vi "Test App Error Handler is Configured Process Added before Start.vi"(8 "error in (no error)":errorcluster, 11 "Rig Test In":refnum<class "Application Dev Test.lvclass">) -> (0 "error out":errorcluster, 3 "Rig Test Out":refnum<class "Application Dev Test.lvclass">)   [LabVIEW 2020, in "Application Dev Test.lvclass"]
uses:
  Application Dev Test.lvclass
  C:/Program Files (x86)/National Instruments/LabVIEW 2020/vi.lib/Astemes/LUnit/Test Case.lvclass
  source/Framework Test Suite/Mock Error Handler/Mock Error Handler.lvclass
  C:/Git/astemes-triarc-framework/source/Framework/Error Handler Interface/Error Handler Interface.lvclass
  source/Framework Test Suite/Mock Process/Mock Process.lvclass
  C:/Git/astemes-triarc-framework/source/Framework/Process/Process.lvclass
  source/Framework/Process/Process.lvclass/Process.ctl
  source/Framework/Application/Application.lvclass/Application.ctl
  <vilib>/Astemes/LUnit/Test Case.lvclass/Test Case.ctl
  <vilib>/Astemes/LUnit/LUnit Assertion Result.lvclass/LUnit Assertion Result.ctl
  <vilib>/Astemes/LUnit/LUnit Test Case Result.lvclass/LUnit Test Case Result.ctl
  <vilib>/Astemes/LUnit/LUnit Method Result.lvclass/LUnit Method Result.ctl
  5ee07f7f-66e8-4a52-8bdc-6cb22f914c3f.vi
  source/Framework/Application/Private/Add Process to Map.vi
  source/Framework/Application/Private/Start Idle Processes if Running.vi
  source/Framework/Application/Private/Throw Error If Process Already in App.vi
  source/Framework/Process/Protected/Messaging/Enqueue Message.vi
  source/Framework/Process/Public/Lifecycle/Get Lifecycle State.vi
  source/Framework/Process/Protected/SubVIs/Set Context.vi
  source/Framework/Application/Private/Retrieve Process from App.vi
  source/Framework/Application/Private/Parse Process Name.vi
  source/Framework/Application/Private/Get Process from Map.vi
  source/Framework/Process/Private/SubVIs/Wait for finish.vi
  source/Framework/Process/Private/SubVIs/Set Lifecycle State.vi
  <vilib>/Astemes/LUnit/Palette/Pass.vi
  <vilib>/Astemes/LUnit/Palette/Fail.vi
  <vilib>/Astemes/LUnit/Compare Variants.vi
  <vilib>/Astemes/LUnit/Describe Comparison.vi
  <vilib>/Astemes/LUnit/Set Assertion Type.vi
  source/Framework/Process/Private/SubVIs/Handle Debug Data.vi
  <vilib>/Utility/error.llb/Clear Errors.vi
  source/Framework/Process/Public/Lifecycle/Leave Process Loop.vi
  source/Framework/Process/Protected/Messaging/Request Message.vi
  <vilib>/AdvancedString/Delimited String to 1D String Array.vi
  <vilib>/Astemes/LUnit/Add test result.vi
  <vilib>/Astemes/LUnit/LUnit Write Passed.vi
  <vilib>/Astemes/LUnit/LUnit Write Message.vi
  <vilib>/Astemes/LUnit/LUnit Write Description.vi
  <vilib>/Astemes/LUnit/Variant to string.vi
  <vilib>/Astemes/LUnit/LUnit Write Assertion Type.vi
  source/Framework/Logging/Log Debug.vi
  <vilib>/AdvancedString/1D String Array to Delimited String.vi
  <vilib>/Utility/High Resolution Relative Seconds.vi
  source/Framework/Process/Private/SubVIs/Enqueue Request Message.vi
  <vilib>/Astemes/LUnit/LUnit Record Assertion Result.vi
  <vilib>/Astemes/LUnit/LUnit Aggregate Assertion Results.vi
  <vilib>/Astemes/LUnit/Assertion Result/LUnit Read Status.vi
  <vilib>/Astemes/LUnit/LUnit Read Message.vi
  <vilib>/Astemes/LUnit/LUnit Read Description.vi
  <vilib>/Astemes/LUnit/Method Result/LUnit Merge Status.vi
  <vilib>/Astemes/LUnit/LUnit Concatenate result strings.vi
  source/Framework/Application/Application.lvclass
  <vilib>/Utility/error.llb/Error Cluster From Error Code.vi
  source/Framework/Process/Public/Read Name.vi
  source/Framework/Process/Private/SubVIs/Wait for Response Message.vi
  <vilib>/Utility/Data Type/Get Type Information.vi
  <vilib>/Utility/LVClass/Get LV Class Name.vi
  source/Framework/Process/Process.lvclass
  <vilib>/Astemes/LUnit/LUnit Assertion Result.lvclass
  source/Framework Test Suite/Support/Test Support.lvlib
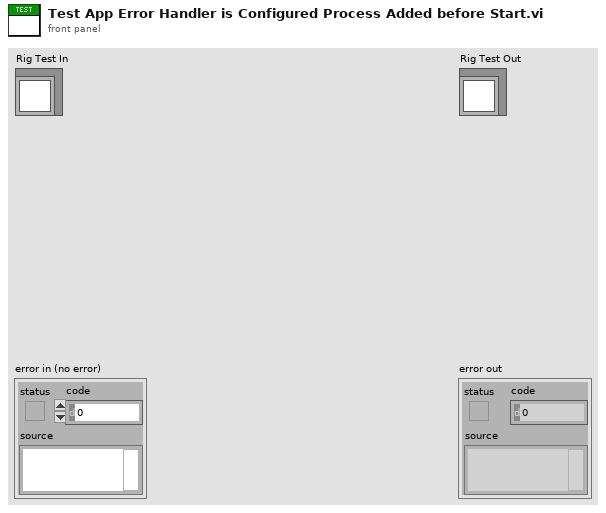
[diagram p1: front panel]
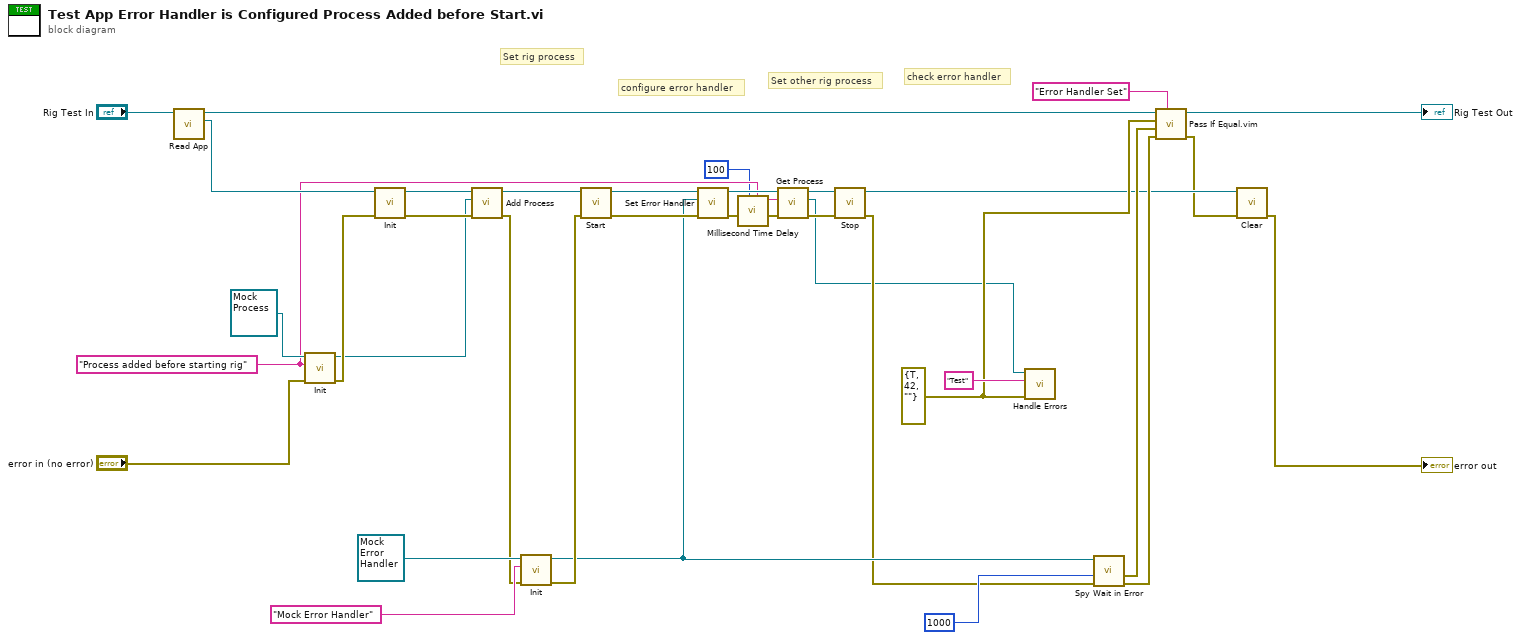
[diagram p0: block diagram]
diagram:
  w17 = errorcluster {"status"=TRUE, "code"=42, "source"=""} ("error in (no error)")
  w5 = "Process added before starting rig" ("Name")
  # "check error handler"
  # "Set other rig process"
  # "configure error handler"
  # "Set rig process"
  n1 = call "Read App.vi"("Application Test In"="Rig Test In") -> ("App out"=w35:refnum<class "Application.lvclass">, "Application Test Out"=w12:refnum<class "Application Dev Test.lvclass">)  [unwired: 8 in, 1 out]
  n2 = call-dynamic "Init.vi"("error in (no error)"="error in (no error)", "Name"=w5, "Mock Process In"=refnum<class "Mock Process.lvclass"> refnum ("Mock Process.lvclass")) -> ("error out"=w26:errorcluster, "Mock Process Out"=w21:refnum<class "Mock Process.lvclass">)  [unwired: 7 in]
  n3 = call-dynamic "Init.vi"("error in (no error)"=w26, "Process In"=w35) -> ("error out"=w24:errorcluster, "Process Out"=w34:refnum<class "Application.lvclass">)  [unwired: 8 in]
  n4 = call "Add Process.vi"("error in (no error)"=w24, "Process"=w21, "Application In"=w34) -> ("error out"=w23:errorcluster, "Application Out"=w25:refnum<class "Application.lvclass">)  [unwired: 7 in]
  n5 = call-dynamic "Init.vi"("error in (no error)"=w23, "Name"="Mock Error Handler", "Mock Error Handler In"=refnum<class "Mock Error Handler.lvclass"> refnum ("Mock Error Handler.lvclass")) -> ("error out"=w29:errorcluster, "Mock Error Handler Out"=w9:refnum<class "Mock Error Handler.lvclass">)  [unwired: 7 in]
  n6 = call "Start.vi"("error in (no error)"=w29, "Process In"=w25) -> ("error out"=w22:errorcluster, "Process Out"=w33:refnum<class "Application.lvclass">)  [unwired: 7 in, 1 out]
  n7 = call "Set Error Handler.vi"("error in (no error)"=w22, "Error Handler"=w9, "Process In"=w33) -> ("error out"=w32:errorcluster, "Process Out"=w7:refnum<class "Application.lvclass">)  [unwired: 7 in]
  n8 = call "Millisecond Time Delay.vi"("milliseconds to wait"=u32 100, "error in (no error)"=w32) -> ("error out"=w2:errorcluster)  [unwired: 7 in]
  n9 = call "Get Process.vi"("error in (no error)"=w2, "Process Name"=w5, "Application In"=w7) -> ("error out"=w8:errorcluster, "App Process"=w3:refnum<class "Process.lvclass">, "Application Out"=w6:refnum<class "Application.lvclass">)  [unwired: 6 in]
  n10 = call "Stop.vi"("error in (no error)"=w8, "Process In"=w6) -> ("error out"=w4:errorcluster, "Process Out"=w13:refnum<class "Application.lvclass">)  [unwired: 7 in, 1 out]
  n11 = call-dynamic "Handle Errors.vi"("error in (no error)"=w17, "Location"="Test", "Process In"=w3) -> ()  [unwired: 7 in, 2 out]
  n12 = call "Spy Wait in Error.vi"("error in (no error)"=w4, "timeout in ms (-1)"=1000, "Mock Error Handler In"=w9) -> ("error out"=w15:errorcluster, "Errors"=w16:errorcluster)  [unwired: 4 in, 3 out]
  n13 = call "Pass If Equal.vim"("Description"="Error Handler Set", "error in (no error)"=w15, "Actual"=w16, "Expected"=w17, "LUnit Test Case In"=w12) -> ("error out"=w10:errorcluster, "LUnit Test Case Out"=→"Rig Test Out":refnum<class "Application Dev Test.lvclass">)  [unwired: 5 in]
  n14 = call-dynamic "Clear.vi"("error in (no error)"=w10, "Application In"=w13) -> ("error out"=→"error out":errorcluster)  [unwired: 9 in]
